vi "Lift State Machine.vi"(8 "Parking Break":T6={"DevStatus"={"status"=FALSE, "code"=0, "source"=""}, "Pneumatics Control Module"=0, "Forward Solenoid Channel"=enum."Invalid", "Reverse Solenoid Channel"=enum."Invalid"}, 9 "Lift Motors":T1[](array[typedef])) -> ()   [LabVIEW 2017]
uses:
  <vilib>/Rock Robotics/WPI/Solenoid/WPI_SolenoidDevRef.ctl
  <vilib>/Rock Robotics/WPI/Solenoid/WPI_SolenoidChannel.ctl
  <vilib>/Rock Robotics/WPI/MotorControl/WPI_MotorControlDeviceRef.ctl
  <vilib>/Rock Robotics/WPI/MotorControl/WPI_MotorControlType.ctl
  <vilib>/Rock Robotics/SystemInterfaces/DIO/FPGA_DIOPWMChannel.ctl
  <vilib>/Rock Robotics/WPI/PWM/WPI_PWMDeadband.ctl
  <vilib>/Rock Robotics/SystemInterfaces/DIO/FPGA_DIOChannel.ctl
  Lift States.ctl
  Parking States.ctl
  <vilib>/Rock Robotics/WPI/Solenoid/WPI_SolenoidValue.ctl
  Robot Global Data.vi
  <vilib>/Rock Robotics/WPI/Solenoid/WPI_SolenoidSetEnum.vi
panel:
  in  "Kp":dbl=0.007
  in  "Scale High Setpoint":dbl=0.03
  in  "Scale Med Setpoint":dbl=0.02
  in  "Scale Low Setpoint":dbl=0.01
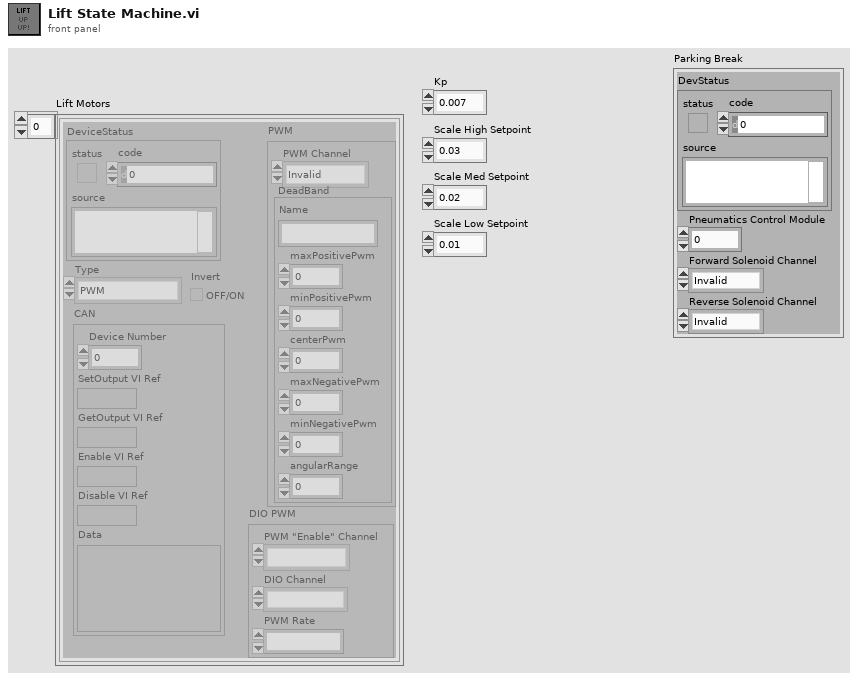
[diagram p1: front panel]
types:
  T1 = typedef "WPI_MotorControlDeviceRef.ctl" = cluster{"DeviceStatus":errorcluster, "Type":T2, "PWM":cluster{"PWM Channel":T3, "DeadBand":T4}, "CAN":cluster{"Device Number":u8, "SetOutput VI Ref":variant, "GetOutput VI Ref":variant, "Enable VI Ref":variant, "Disable VI Ref":variant, "Data":variant}, "Invert":bool, "DIO PWM":cluster{"PWM \"Enable\" Channel":T3, "DIOChannel":T5, "PWM Rate":dbl}}
  T2 = typedef "WPI_MotorControlType.ctl" = enum16{"PWM", "CAN", "DIO PWM"}
  T3 = typedef "FPGA_DIOPWMChannel.ctl" = enum8{"PWM 0", "PWM 1", "PWM 2", "PWM 3", "PWM 4", "PWM 5", "PWM 6", "PWM 7", "PWM 8", "PWM 9", "PWM MXP 0", "PWM MXP 1", "PWM MXP 2", "PWM MXP 3", "PWM MXP 4", "PWM MXP 5", "PWM MXP 6", "PWM MXP 7", "PWM MXP 8", "PWM MXP 9", "Invalid"}
  T4 = typedef "WPI_PWMDeadband.ctl" = cluster{"Name":string, "maxPositivePwm":i32, "minPositivePwm":i32, "centerPwm":i32, "maxNegativePwm":i32, "minNegativePwm":i32, "angularRange":u16}
  T5 = typedef "FPGA_DIOChannel.ctl" = enum8{"DIO 0", "DIO 1", "DIO 2", "DIO 3", "DIO 4", "DIO 5", "DIO 6", "DIO 7", "DIO 8", "DIO 9", "DIO MXP 0", "DIO MXP 1", "DIO MXP 2", "DIO MXP 3", "DIO MXP 4", "DIO MXP 5", "DIO MXP 6", "DIO MXP 7", "DIO MXP 8", "DIO MXP 9", "DIO MXP 10", "DIO MXP 11", "DIO MXP 12", "DIO MXP 13", "DIO MXP 14", "DIO MXP 15", "SPI Port CS1", "SPI Port CS2", "SPI Port CS3", "SPI Port MISO", "SPI Port MOSI", "Invalid"}
  T6 = typedef "WPI_SolenoidDevRef.ctl" = cluster{"DevStatus":errorcluster, "Pneumatics Control Module":u8, "Forward Solenoid Channel":T7, "Reverse Solenoid Channel":T7}
  T7 = typedef "WPI_SolenoidChannel.ctl" = enum8{"Solenoid 0", "Solenoid 1", "Solenoid 2", "Solenoid 3", "Solenoid 4", "Solenoid 5", "Solenoid 6", "Solenoid 7", "Invalid"}
  T8 = typedef "WPI_SolenoidValue.ctl" = enum16{"Off", "On", "Forward", "Reverse"}
  T9 = typedef "Parking States.ctl" = enum16{"Not Parked", "Parked"}
  T10 = typedef "Lift States.ctl" = enum16{"Manual", "Scale Low", "Scale Middle", "Scale High"}
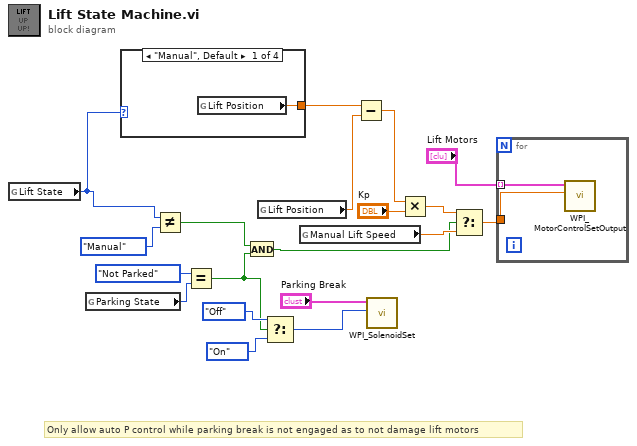
[diagram p0: block diagram]
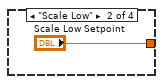
[diagram p2: hidden frame]
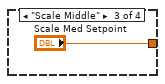
[diagram p3: hidden frame]
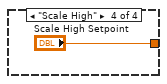
[diagram p4: hidden frame]
diagram:
  # "Only allow auto P control while parking break is not engaged as to not damage lift motors"
  n1 = global read "Robot Global Data.vi" "Lift State"() -> (w8:T10)
  n2 = global read "Robot Global Data.vi" "Parking State"() -> (w12:T9)
  n3 = case shown="\"Manual\", Default" w8 {
    tunnel: [w20 "Scale Low Setpoint" "Scale Med Setpoint" "Scale High Setpoint"] -> w14
    frame "Manual", Default {
      n4 = global read "Robot Global Data.vi" "Lift Position"() -> (w20:dbl)
    }
    frame "Scale Low" {
    }
    frame "Scale Middle" {
    }
    frame "Scale High" {
    }
  }
  n5 = Not Equal?(x=w8, y=Lift_States."Manual") -> (x != y?=w10:bool)
  n6 = Equal?(x=Parking_States."Not Parked", y=w12) -> (x = y?=w4:bool)
  n7 = And(x=w10, y=w4) -> (x .and. y?=w9:bool)
  n8 = global read "Robot Global Data.vi" "Lift Position"() -> (w13:dbl)
  n9 = Select(t=WPI_SolenoidValue."Off" ("Value"), s=w4, f=WPI_SolenoidValue."On" ("Value")) -> (s? t:f=w3:T8)
  n10 = global read "Robot Global Data.vi" "Manual Lift Speed"() -> (w15:dbl)
  n11 = Subtract(x=w14, y=w13) -> (x-y=w16:dbl)
  n12 = call-poly <vilib>:"WPI_SolenoidSet.vi"("Value"=w3, "SolenoidDevRef"="Parking Break") -> ()  [unwired: 8 in, 2 out]
  n13 = Multiply(x=w16, y="Kp") -> (x*y=w18:dbl)
  n14 = Select(t=w18, s=w9, f=w15) -> (s? t:f=w2:dbl)
  n15 = for {
    tunnel: w2 -> [w25]
    tunnel: "Lift Motors" -> [w24] mode=indexing
    n16 = call <vilib>:"WPI_MotorControlSetOutput.vi"("Output"=w25, "MotorControlDevRef"=w24) -> ()  [unwired: 7 in, 3 out]
  }
